vi "Legendre Polynomial_Standard (1D).vi"(8 "m":i32, 9 "n":i32, 11 "X":dbl[](array[numeric])) -> (3 "Pnm(X)":dbl[](array[numeric]))   [LabVIEW 2017, in "NI_AAL_Polynomial.lvlib"]
uses:
  <vilib>/Analysis/NI_AAL_Polynomial.lvlib
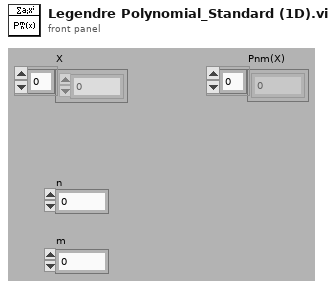
[diagram p1: front panel]
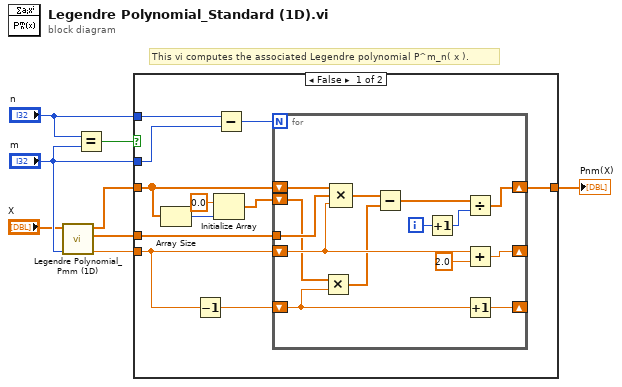
[diagram p0: block diagram]
diagram:
  # "This vi computes the associated Legendre polynomial P^m_n( x )."
  n1 = call <vilib>:"Legendre Polynomial_Pmm (1D).vi"("m"="m", "X In"="X") -> ("2m+1"=w4:dbl, "X Out"=w3:dbl[], "Pmm(X)"=w6:dbl[])  [unwired: 6 out]
  n2 = Equal?(x="n", y="m") -> (x = y?=w8:bool)
  n3 = case shown="False" w8 {
    tunnel: w6 -> [w10 w34]
    tunnel: w4 -> [w14 _]
    tunnel: "m" -> [w17 _]
    tunnel: "n" -> [w18 _]
    tunnel: [w19 w34] -> w2
    tunnel: w3 -> [w15 _]
    frame False {
      n4 = Array Size(array=w10) -> (size(s)=w12:i32)
      n5 = Decrement(x=w14) -> (x-1=w13:dbl)
      n6 = Initialize Array(0.0 ("P^m_m"), w12) -> (w9:dbl[])
      n7 = Subtract(x=w18, y=w17) -> (x-y=w16:i32)
      n8 = for {
        N: w16 -> [_]
        shift-right: [w23] -> w19
        shift-left: w10 -> [w28]
        shift-left: w9 -> [w26]
        shift-right: [w33] -> _
        shift-left: w14 -> [w29]
        tunnel: w15 -> [w30]
        shift-right: [w31] -> _
        shift-left: w13 -> [w27]
        i -> [w21]
        n9 = Multiply(x=w26, y=w27) -> (x*y=w24:dbl[])
        n10 = Compound Arithmetic op=MULTIPLY(w28, w30, w29) -> (w25:dbl[])
        n11 = Subtract(x=w25, y=w24) -> (x-y=w22:dbl[])
        n12 = Increment(x=w21) -> (x+1=w20:i32)
        n13 = Divide(x=w22, y=w20) -> (x/y=w23:dbl[])
        n14 = Add(x=w29, y=2.0 ("x")) -> (x+y=w33:dbl)
        n15 = Increment(x=w27) -> (x+1=w31:dbl)
      }
    }
    frame True {
    }
  }
  "Pnm(X)" <- w2
